vi "niRFUtil FTW Compute RBW Response Info.vi"(0 "Type":T1=enum."Gaussian", 5 "Center Frequency (Hz)":dbl format="%^.2e", 7 "Bandwidth (Hz)":T2 format="%^.3e", 9 "df (Hz)":dbl format="%^.2e", 11 "Minimum Selectivity (dB)":dbl=70.0 format="%.2f") -> (4 "Start Frequency (Hz)":sgl format="%.2f")   [LabVIEW 2015, in "niRFUtil.lvlib"]
doc: "(c) Copyright 2006, National Instruments, Inc. This VI may not be duplicated, sold, or distributed without written consent from National Instruments."
uses:
  niRFUtil.lvlib
  Includes/niRFUtil INC RBW Filter Bandwidth.ctl
  Includes/niRFUtil INC RBW Filter Type (Freq Domain).ctl
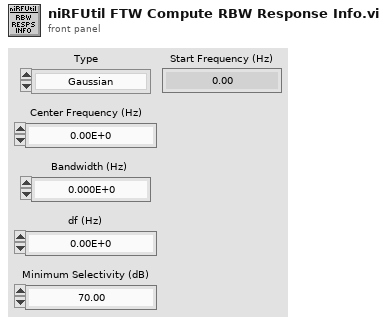
[diagram p1: front panel]
types:
  T1 = typedef "niRFUtil.lvlib/niRFUtil INC RBW Filter Type (Freq Domain).ctl" = enum16{"FFT Based", "Gaussian", "Flat", "Synch Tuned - 4", "Synch Tuned - 5"}
  T2 = typedef "niRFUtil.lvlib/niRFUtil INC RBW Filter Bandwidth.ctl" = dbl
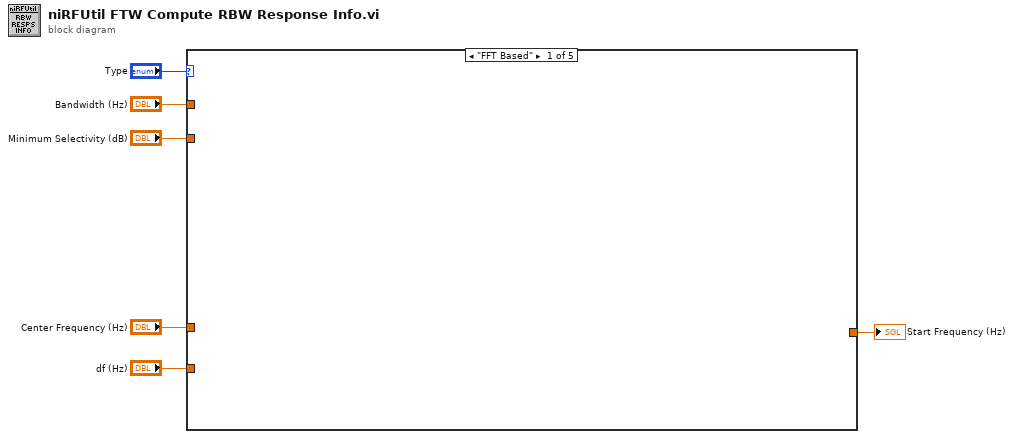
[diagram p0: block diagram]
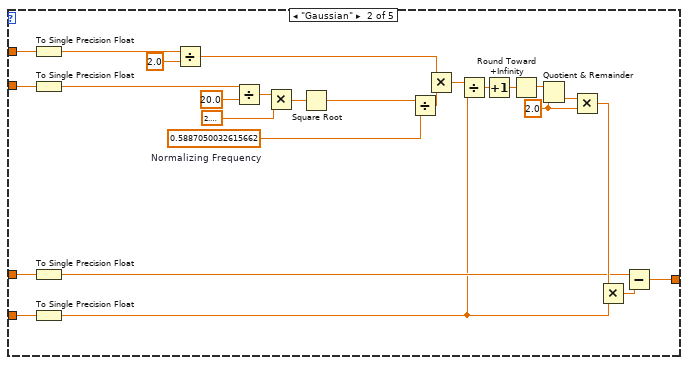
[diagram p2: hidden frame]
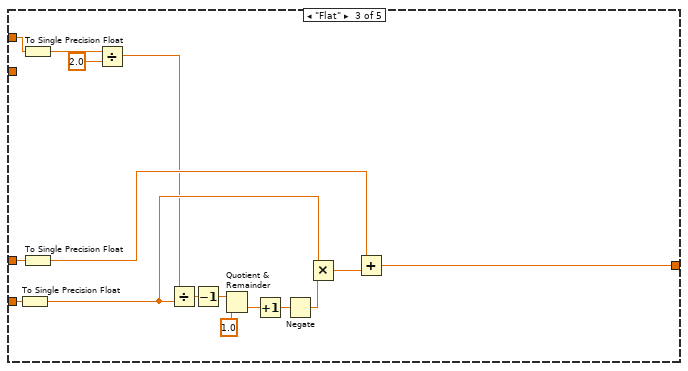
[diagram p3: hidden frame]
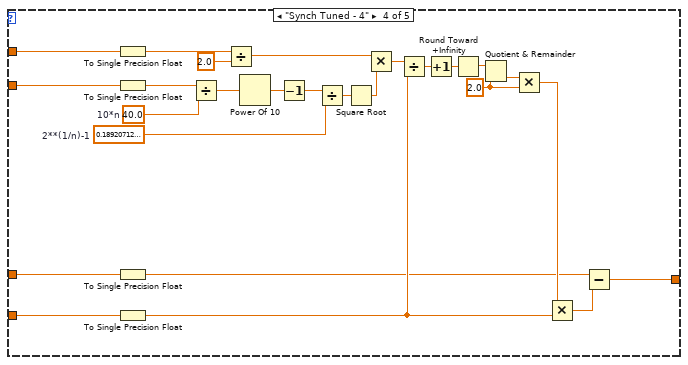
[diagram p4: hidden frame]
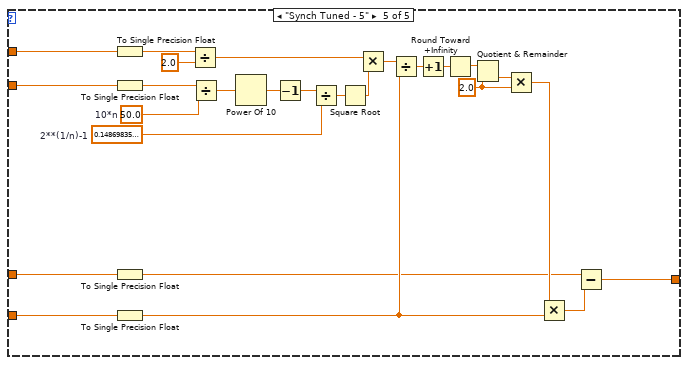
[diagram p5: hidden frame]
diagram:
  n1 = case shown="\"FFT Based\"" "Type" {
    tunnel: "Center Frequency (Hz)" -> [_ w18 w43 w58 w84]
    tunnel: "Bandwidth (Hz)" -> [_ w20 w44 w60 w86]
    tunnel: "df (Hz)" -> [_ w17 w42 w57 w83]
    tunnel: "Minimum Selectivity (dB)" -> [_ w19 _ w59 w85]
    tunnel: [_ w16 w41 w61 w87] -> w1
    frame "FFT Based" {
    }
    frame "Gaussian" {
      w25 = sgl 2.0 ("y")
      w29 = sgl 0.588705  # Normalizing Frequency
      n2 = To Single Precision Float(number=w20) -> (single precision float=w9:sgl)
      n3 = To Single Precision Float(number=w19) -> (single precision float=w15:sgl)
      n4 = To Single Precision Float(number=w18) -> (single precision float=w22:sgl)
      n5 = To Single Precision Float(number=w17) -> (single precision float=w21:sgl)
      n6 = Divide(x=w9, y=sgl 2.0) -> (x/y=w7:sgl)
      n7 = Divide(x=w15, y=sgl 20.0) -> (x/y=w13:sgl)
      n8 = Multiply(x=w13, y=sgl 2.3025851) -> (x*y=w11:sgl)
      n9 = Square Root(x=w11) -> (sqrt(x)=w10:sgl)
      n10 = Divide(x=w10, y=w29) -> (x/y=w30:sgl)
      n11 = Multiply(x=w7, y=w30) -> (x*y=w32:sgl)
      n12 = Divide(x=w32, y=w21) -> (x/y=w28:sgl)
      n13 = Increment(x=w28) -> (x+1=w23:sgl)
      n14 = Round Toward +Infinity(x=w23) -> (ceil(x): smallest int >= x=w27:sgl)
      n15 = Quotient & Remainder(x=w27, y=w25) -> (floor(x/y)=w26:sgl)  [unwired: 1 out]
      n16 = Multiply(x=w26, y=w25) -> (x*y=w24:sgl)
      n17 = Multiply(x=w24, y=w21) -> (x*y=w31:sgl)
      n18 = Subtract(x=w22, y=w31) -> (x-y=w16:sgl)
    }
    frame "Flat" {
      n19 = To Single Precision Float(number=w42) -> (single precision float=w36:sgl)
      n20 = To Single Precision Float(number=w44) -> (single precision float=w35:sgl)
      n21 = To Single Precision Float(number=w43) -> (single precision float=w37:sgl)
      n22 = Divide(x=w35, y=sgl 2.0) -> (x/y=w33:sgl)
      n23 = Divide(x=w33, y=w36) -> (x/y=w48:sgl)
      n24 = Decrement(x=w48) -> (x-1=w45:sgl)
      n25 = Quotient & Remainder(x=w45, y=sgl 1.0) -> (floor(x/y)=w40:sgl)  [unwired: 1 out]
      n26 = Increment(x=w40) -> (x+1=w39:sgl)
      n27 = Negate(x=w39) -> (-x=w38:sgl)
      n28 = Multiply(x=w36, y=w38) -> (x*y=w46:sgl)
      n29 = Add(x=w37, y=w46) -> (x+y=w41:sgl)
    }
    frame "Synch Tuned - 4" {
      w56 = sgl 0.18920712  # 2**(1/n)-1
      w55 = sgl 40.0  # 10*n
      w70 = sgl 2.0 ("y")
      n30 = To Single Precision Float(number=w60) -> (single precision float=w51:sgl)
      n31 = To Single Precision Float(number=w59) -> (single precision float=w64:sgl)
      n32 = To Single Precision Float(number=w58) -> (single precision float=w65:sgl)
      n33 = To Single Precision Float(number=w57) -> (single precision float=w66:sgl)
      n34 = Divide(x=w64, y=w55) -> (x/y=w53:sgl)
      n35 = Divide(x=w51, y=sgl 2.0) -> (x/y=w50:sgl)
      n36 = Power Of 10(x=w53) -> (10^x=w54:sgl)
      n37 = Decrement(x=w54) -> (x-1=w52:sgl)
      n38 = Divide(x=w52, y=w56) -> (x/y=w63:sgl)
      n39 = Square Root(x=w63) -> (sqrt(x)=w62:sgl)
      n40 = Multiply(x=w50, y=w62) -> (x*y=w74:sgl)
      n41 = Divide(x=w74, y=w66) -> (x/y=w68:sgl)
      n42 = Increment(x=w68) -> (x+1=w69:sgl)
      n43 = Round Toward +Infinity(x=w69) -> (ceil(x): smallest int >= x=w72:sgl)
      n44 = Quotient & Remainder(x=w72, y=w70) -> (floor(x/y)=w71:sgl)  [unwired: 1 out]
      n45 = Multiply(x=w71, y=w70) -> (x*y=w67:sgl)
      n46 = Multiply(x=w67, y=w66) -> (x*y=w73:sgl)
      n47 = Subtract(x=w65, y=w73) -> (x-y=w61:sgl)
    }
    frame "Synch Tuned - 5" {
      w82 = sgl 0.14869836  # 2**(1/n)-1
      w81 = sgl 50.0  # 10*n
      w96 = sgl 2.0 ("y")
      n48 = To Single Precision Float(number=w86) -> (single precision float=w77:sgl)
      n49 = To Single Precision Float(number=w85) -> (single precision float=w90:sgl)
      n50 = To Single Precision Float(number=w84) -> (single precision float=w91:sgl)
      n51 = To Single Precision Float(number=w83) -> (single precision float=w92:sgl)
      n52 = Divide(x=w77, y=sgl 2.0) -> (x/y=w75:sgl)
      n53 = Divide(x=w90, y=w81) -> (x/y=w80:sgl)
      n54 = Power Of 10(x=w80) -> (10^x=w79:sgl)
      n55 = Decrement(x=w79) -> (x-1=w78:sgl)
      n56 = Divide(x=w78, y=w82) -> (x/y=w89:sgl)
      n57 = Square Root(x=w89) -> (sqrt(x)=w88:sgl)
      n58 = Multiply(x=w75, y=w88) -> (x*y=w100:sgl)
      n59 = Divide(x=w100, y=w92) -> (x/y=w94:sgl)
      n60 = Increment(x=w94) -> (x+1=w95:sgl)
      n61 = Round Toward +Infinity(x=w95) -> (ceil(x): smallest int >= x=w98:sgl)
      n62 = Quotient & Remainder(x=w98, y=w96) -> (floor(x/y)=w97:sgl)  [unwired: 1 out]
      n63 = Multiply(x=w97, y=w96) -> (x*y=w93:sgl)
      n64 = Multiply(x=w93, y=w92) -> (x*y=w99:sgl)
      n65 = Subtract(x=w91, y=w99) -> (x-y=w87:sgl)
    }
  }
  "Start Frequency (Hz)" <- w1
